vi "Detect Goertzel.vi"(0 "Signal":dbl[](array[numeric]), 1 "frequency":dbl) -> (7 "Numeric":dbl)   [LabVIEW 2014]
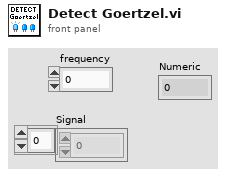
[diagram p1: front panel]
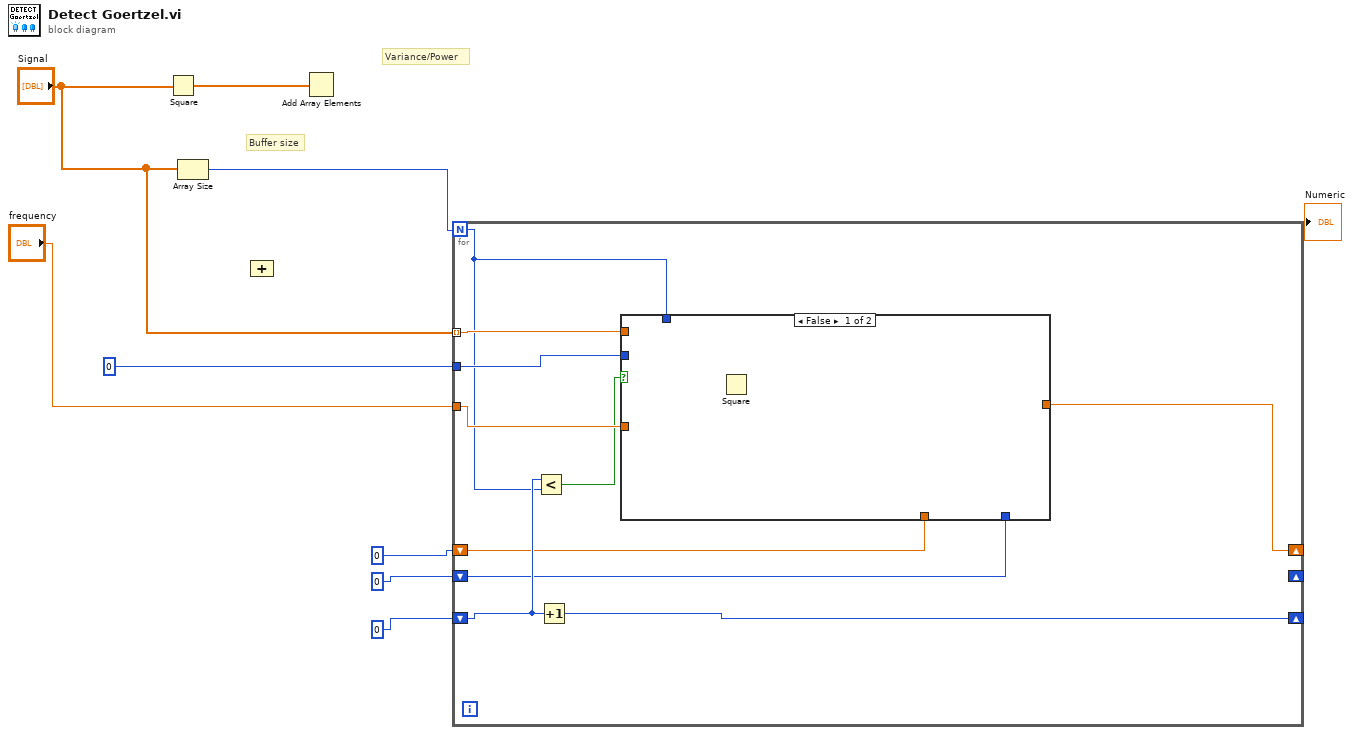
[diagram p0: block diagram]
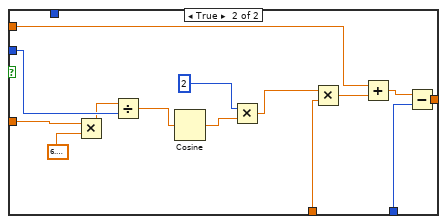
[diagram p2: hidden frame]
diagram:
  # "Buffer size"
  # "Variance/Power"
  n1 = Square(x="Signal") -> (x^2=w9:dbl[])
  n2 = Array Size(array="Signal") -> (size(s)=w7:i32)
  n3 = Compound Arithmetic op=ADD() -> ()  [unwired: 2 in, 1 out]
  n4 = Add Array Elements(numeric array=w9) -> (sum=w8:dbl)
  n5 = for {
    N: w7 -> [w10]
    tunnel: "frequency" -> [w17]
    shift-right: [w12] -> _
    shift-left: 0 -> [w15]
    shift-right: _ -> [_]
    shift-left: 0 -> [w14]
    tunnel: "Signal" -> [w13] mode=indexing
    shift-right: [w19] -> _
    shift-left: 0 -> [w18]
    tunnel: 0 -> [w16]
    n6 = Less?(x=w18, y=w10) -> (x < y?=w11:bool)
    n7 = Increment(x=w18) -> (x+1=w19:i32)
    n8 = case shown="False" w11 {
      tunnel: w17 -> [_ w27]
      tunnel: w16 -> [_ w26]
      tunnel: w15 -> [_ w23]
      tunnel: w14 -> [_ w22]
      tunnel: w13 -> [_ w21]
      tunnel: [_ w20] -> w12
      tunnel: w10 -> [_ _]
      frame False {
        n9 = Square() -> ()  [unwired: 1 in, 1 out]
      }
      frame True {
        n10 = Multiply(x=w27, y=6.283185307179586) -> (x*y=w25:dbl)
        n11 = Divide(x=w25, y=w26) -> (x/y=w24:dbl)
        n12 = Cosine(x=w24) -> (cos(x)=w28:dbl)
        n13 = Multiply(x=2, y=w28) -> (x*y=w31:dbl)
        n14 = Multiply(x=w31, y=w23) -> (x*y=w32:dbl)
        n15 = Add(x=w21, y=w32) -> (x+y=w33:dbl)
        n16 = Subtract(x=w33, y=w22) -> (x-y=w20:dbl)
      }
    }
  }
